vi "FillTable.vi"(11 "Array":string[][](array[string])) -> (3 "Table Control":string[][](table))   [LabVIEW 2023]
panel:
  out "2D String Array":string[][](array[string])
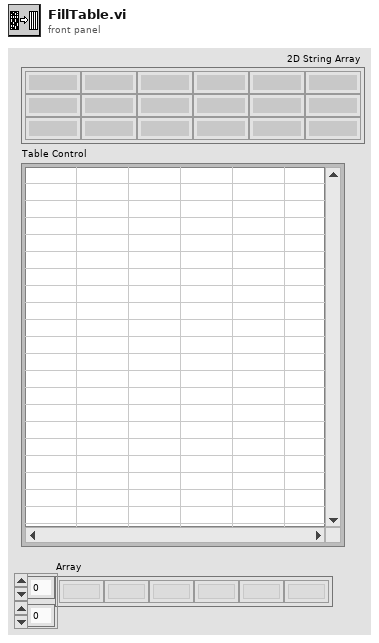
[diagram p1: front panel]
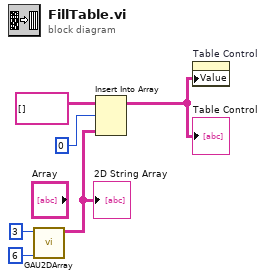
[diagram p0: block diagram]
diagram:
  n1 = call "GAU2DArray.vi"("Colums"=6, "Rows"=3) -> ("2D String Array"=w1:string[][])  [unwired: 7 in, 2 out]
  "2D String Array" <- w1
  n2 = Insert Into Array "Insert Into Array"(array=string[][] [], index (row)=0 ("index"), new element=w1) -> (w5:string[][])  [unwired: 1 in]
  "Table Control" <- w5
  n3 = property on="Table Control" class="Tbl (strict)"("Value"=w5) -> ()  [unwired: 2 in, 2 out]
